vi "kernel.vi"(10 "size":i32, 11 "sigma":dbl) -> ()   [LabVIEW 2013]
panel:
  out "Array":dbl[][](array[numeric])
  in  "Text Ring":u16(ring) items=["circle", "gauss", "sobel", "laplace", "log", ""]
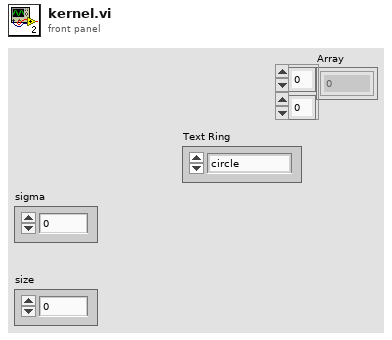
[diagram p1: front panel]
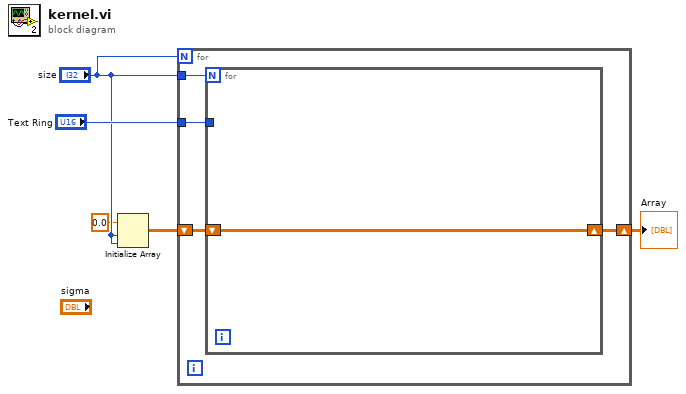
[diagram p0: block diagram]
diagram:
  n1 = Initialize Array(0.0 ("element"), "size", "size") -> (w3:dbl[][])
  n2 = for {
    N: "size" -> [_]
    tunnel: "Text Ring" -> [w9]
    tunnel: "size" -> [w8]
    shift-right: [w6] -> w1
    shift-left: w3 -> [w7]
    n3 = for {
      N: w8 -> [_]
      tunnel: w9 -> [_]
      shift-right: [w10] -> w6
      shift-left: w7 -> [w10]
    }
  }
  "Array" <- w1
